vi "Return string before whitespace or comma.vi"(8 "error in (no error)":errorcluster, 11 "String":string) -> (0 "error out":errorcluster, 3 "Extracted string":string)   [LabVIEW 2013]
doc: "Return string contents until whitespace or comma or end of string starting at the first char"
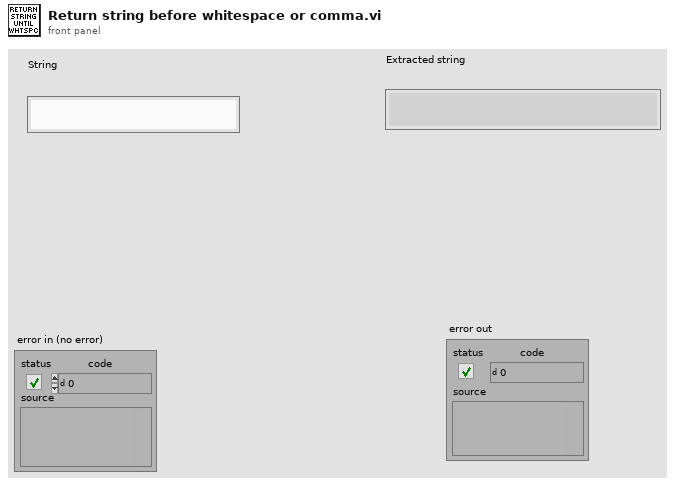
[diagram p1: front panel]
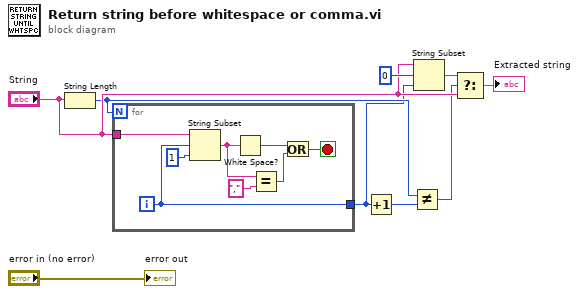
[diagram p0: block diagram]
diagram:
  n1 = String Length(string="String") -> (length=w5:i32)
  n2 = for {
    N: w5 -> [_]
    tunnel: "String" -> [w17]
    tunnel: [w15] -> w2
    i -> [w15]
    stop <- w10 stop-if-true
    n3 = String Subset(string=w17, offset (0)=w15, length (rest)=1 ("length (rest)")) -> (substring=w14:string)
    n4 = White Space?(1:w14) -> (0:w12:bool)
    n5 = Equal?(x=w14, y=",") -> (x = y?=w11:bool)
    n6 = Or(x=w12, y=w11) -> (x .or. y?=w10:bool)
  }
  n7 = Increment(x=w2) -> (x+1=w1:i32)
  n8 = Not Equal?(x=w5, y=w1) -> (x != y?=w4:bool)
  n9 = String Subset(string="String", offset (0)=0, length (rest)=w2) -> (substring=w7:string)
  n10 = Select(t=w7, s=w4, f="String") -> (s? t:f=→"Extracted string":string)
  "error out" <- "error in (no error)"
